vi "oa_Order Magnitude dB Processing (1 Channel).vi"(9 "dB on? (T)":bool=TRUE, 10 "even angle channel info":T1={"channel name"="", "description"="", " channel info"={"sensor sensitivity"=1000.0, "engineering units"=1, "dB reference"=1.0, "custom label"="EU", "weighting filter"=0, "pregain"=0.0}} {"channel info"."pregain" format="%.2f"; "channel info"."weighting filter" items=["Linear", "A-weighting", "B-weighting", "C-weighting", "ITU-R 468-4", "Dolby", "CCITT", "C-message", "Wb", "Wc", "Wd", "We", "Wf", "Wh", "Wj", "Wk", "Wm", "AES17 20 kHz lowpass", "AES17 40 kHz lowpass", "AES17 20 kHz highpass", "AES17 40 kHz highpass"]; "channel info"."dB reference" format="%^.1e"; "channel info"."engineering units" items=["custom..."=0, "V"=1, "A"=21, "C"=30, "pC"=31, "s"=32, "-"=29, "Pa"=2, "N"=20, "g"=3, "m/s^2"=4, "m/s"=5, "m"=6, "mm/s"=12, "mm"=13, "micron/s"=14, "micron"=15, "in/s^2"=7, "in/s"=8, "in"=9, "mil/s"=10, "mil"=11, "rad/s^2"=16, "rad/s"=17, "rad"=18, "deg/s^2"=26, "deg/s"=27, "deg"=28, "RPM"=22, "cycle/s^2"=23, "Hz"=24, "cycle"=25, "strain"=19]; "channel info"."sensor sensitivity" format="%#_5f"}, 11 "magnitudes":T5(array[cluster]) {"magnitude" format="%.2f"; "time/rev/rpm" format="%.2f"}) -> (3 "magnitudes dB":T5(array[cluster]) {"magnitude" format="%.2f"; "time/rev/rpm" format="%.2f"})   [LabVIEW 2017, in "SoundVib_Resampling.lvlib"]
uses:
  <vilib>/addons/Sound and Vibration/Order Analysis/Resample Order Tracking/SoundVib_Resampling.lvlib
  <vilib>/addons/_NISVFA/_Shared subVIs/Controls/svc_Resampled Channel Info.ctl
  <vilib>/addons/_NISVFA/_Shared subVIs/Controls/svc_Channel Info.ctl
  <vilib>/addons/_NISVFA/_Shared subVIs/Controls/svc_Engineering Units Text Ring.ctl
  <vilib>/addons/_NISVFA/_Shared subVIs/Controls/svc_Weighting Filter Text Ring.ctl
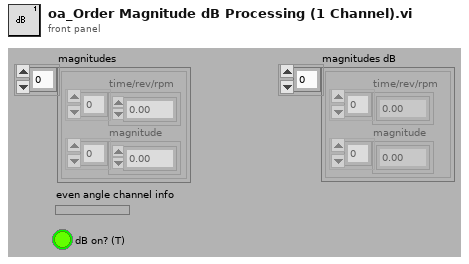
[diagram p1: front panel]
types:
  T1 = typedef "svc_Resampled Channel Info.ctl" = cluster{"channel name":string, "description":string, " channel info":T2}
  T2 = typedef "svc_Channel Info.ctl" = cluster{"sensor sensitivity":dbl, "engineering units":T3, "dB reference":dbl, "custom label":string, "weighting filter":T4, "pregain":dbl}
  T3 = typedef "svc_Engineering Units Text Ring.ctl" = u16
  T4 = typedef "svc_Weighting Filter Text Ring.ctl" = u16
  T5 = cluster{"time/rev/rpm":dbl[], "magnitude":dbl[]}[]
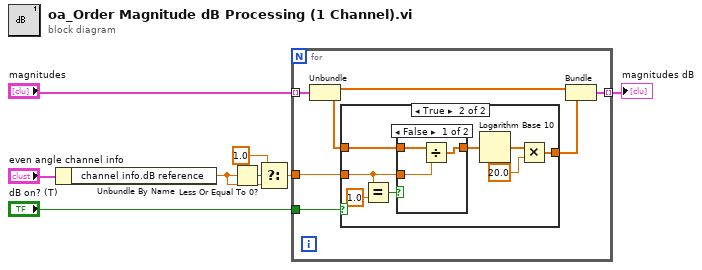
[diagram p0: block diagram]
diagram:
  n1 = Unbundle By Name("even angle channel info") -> ("channel info.dB reference"=w2:dbl)
  n2 = Less Or Equal To 0?(x=w2) -> (x <= 0?=w4:bool)
  n3 = Select(t=1.0, s=w4, f=w2) -> (s? t:f=w1:dbl)
  n4 = for {
    tunnel: "magnitudes" -> [w15] mode=indexing
    tunnel: [w13] -> w7 mode=indexing
    tunnel: "dB on? (T)" -> [w12]
    tunnel: w1 -> [w9]
    n5 = Unbundle(w15) -> ("time/rev/rpm"=w14:dbl[], "magnitude"=w11:dbl[])
    n6 = case shown="True" w12 {
      tunnel: w11 -> [w16 w19]
      tunnel: [w16 w22] -> w10
      tunnel: w9 -> [_ w17]
      frame False {
      }
      frame True {
        n7 = Equal?(x=w17, y=1.0) -> (x = y?=w20:bool)
        n8 = case shown="False" w20 {
          tunnel: w19 -> [w27 w28]
          tunnel: [w25 w28] -> w18
          tunnel: w17 -> [w26 _]
          frame False {
            n9 = Divide(x=w27, y=w26) -> (x/y=w25:dbl[])
          }
          frame True {
          }
        }
        n10 = Logarithm Base 10(1:w18) -> (0:w24:dbl[])
        n11 = Multiply(x=w24, y=20.0) -> (x*y=w22:dbl[])
      }
    }
    n12 = Bundle("time/rev/rpm"=w14, "magnitude"=w10) -> (w13:cluster{"time/rev/rpm":dbl[], "magnitude":dbl[]})  [unwired: 1 in]
  }
  "magnitudes dB" <- w7
